vi "BotSpeak_GetVar.vi"(2 "Variable In":string="power", 3 "Bot Settings":T1) -> (0 "response":string, 1 "Bot Settings out":T1)   [LabVIEW 2012]
doc: "Retrieves the value of \"Variable in\" and returns that as \"value\". If the value is a number, this VI also returns that value in double format as \"number\"."
uses:
  <userlib>/botspeak/VIs/Direct/BotSpeak_Control.ctl
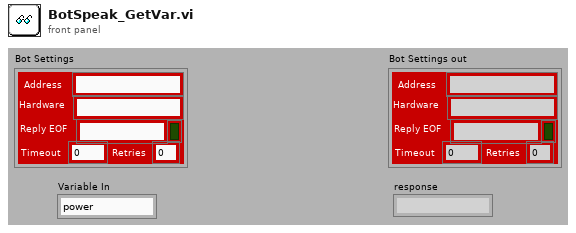
[diagram p1: front panel]
types:
  T1 = typedef "BotSpeak_Control.ctl" = cluster{"Address":string, "Reply EOF":string, "Hardware":string, "Retries":i8, "Timeout":i32, "Open?":bool}
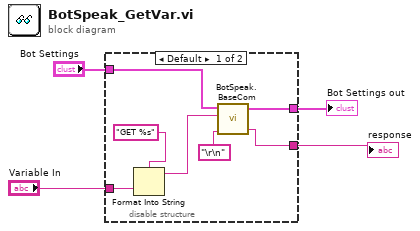
[diagram p0: block diagram]
diagram:
  n1 = disable-structure shown="Default" {
    disable-tunnel: "Bot Settings" -> [w9 _]
    disable-tunnel: [w8 _] -> w3
    disable-tunnel: [w7 _] -> w2
    disable-tunnel: "Variable In" -> [w6 _]
    frame condition #0 (active) {
      n2 = Format Into String(format string="GET %s" ("command"), w6) -> (resulting string=w11:string)  [unwired: 2 in, 1 out]
      n3 = call <userlib>:"BotSpeak.BaseCom.vi"("Termination"="\r\n", "command"=w11, "Bot Settings in"=w9) -> ("response"=w7:string, "Bot Settings out"=w8:T1)  [unwired: 2 in]
    }
    frame condition #1 {
    }
  }
  "Bot Settings out" <- w3
  "response" <- w2
